vi "Read.vi"(8 "error in (no error)":errorcluster, 11 "Add in":refnum<class "AbsFunc_Two Term_Time.lvclass">) -> (0 "error out":errorcluster, 2 "Numeric":T1, 3 "Add out":refnum<class "AbsFunc_Two Term_Time.lvclass">)   [LabVIEW 2021, in "AbsFunc_Two Term_Time.lvclass"]
uses:
  AbsFunc_Two Term_Time.lvclass
  Support/Data Type.ctl
  AbsFunc_Two Term_Time.lvclass/AbsFunc_Two Term_Time.ctl
  Abs_Types/Time/Abs_Time.lvclass
  Abs_Types/Numeric/Abs_Numeric.lvclass
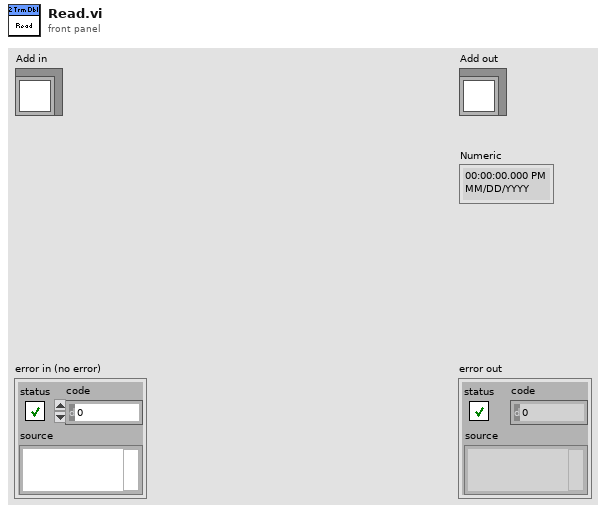
[diagram p1: front panel]
types:
  T1 = typedef "AbsFunc_Two Term_Time.lvclass/Data Type.ctl" = timestamp
  T2 = typedef "AbsFunc_Two Term_Time.lvclass/Abstract Type.ctl" = refnum<class "Abs_Time.lvclass">
  T3 = typedef "Abs_Time.lvclass/Type.ctl" = timestamp
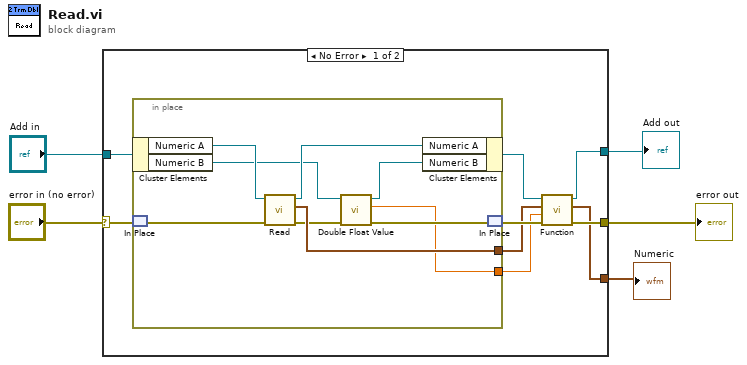
[diagram p0: block diagram]
diagram:
  n1 = case shown="No Error" "error in (no error)" {
    selector: "error in (no error)" -> [w13 w24]
    tunnel: "Add in" -> [w14 w25]
    tunnel: [w10 w25] -> w3
    tunnel: [w9 w24] -> w2
    tunnel: [w6 _] -> w1
    frame No Error {
      n2 = in-place {
        in-place-border: [w20] -> w8
        in-place-border: [w15] -> w7
        n3 = in-place-cluster #1(w14) -> ("Numeric A"=w23:T2, "Numeric B"=w19:refnum<class "Abs_Numeric.lvclass">)
        n4 = in-place-match #2(w13) -> (w22:errorcluster)
        n5 = call-dynamic "Read.vi"("error in (no error)"=w22, "Double Float.lvclass_340760 in"=w23) -> ("error out"=w17:errorcluster, "Value"=w20:T3, "Double Float.lvclass_340760 out"=w21:T2)  [unwired: 7 in]
        n6 = call-dynamic "Double Float Value.vi"("error in (no error)"=w17, "Numeric in"=w19) -> ("error out"=w16:errorcluster, "Double"=w15:dbl, "Numeric out"=w18:refnum<class "Abs_Numeric.lvclass">)  [unwired: 7 in]
        n7 = in-place-cluster #1("Numeric A"=w21, "Numeric B"=w18) -> (w11:refnum<class "AbsFunc_Two Term_Time.lvclass">)
        n8 = in-place-match #2(w16) -> (w12:errorcluster)
      }
      n9 = call-dynamic "Function.vi"("error in (no error)"=w12, "Numeric B"=w7, "Numeric A"=w8, "Two Terminal in"=w11) -> ("error out"=w9:errorcluster, "Result"=w6:T1, "Two Terminal out"=w10:refnum<class "AbsFunc_Two Term_Time.lvclass">)  [unwired: 5 in]
    }
    frame Error {
    }
  }
  "error out" <- w2
  "Add out" <- w3
  "Numeric" <- w1
